vi "SaveImageAndDATA.vi"(6 "Array":dbl[][](array[numeric]), 7 "new picture":picture, 9 "Info":string, 10 "file name":string, 11 "folder":path) -> ()   [LabVIEW 2011]
uses:
  <vilib>/Utility/file.llb/Write To Spreadsheet File (DBL).vi
panel:
  out "before substring":string
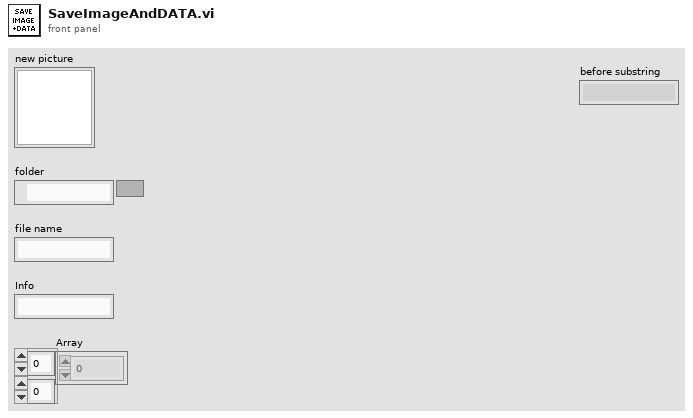
[diagram p1: front panel]
types:
  T1 = enum16{"open", "replace", "create", "open or create", "replace or create", "replace or create with confirmation"}
  T2 = typedef "imagedata.ctl" = cluster{"image type":i32, "image depth":i32, "image":u8[], "mask":u8[], "colors":u32[], "Rectangle":cluster{"left":i16, "top":i16, "right":i16, "bottom":i16}}
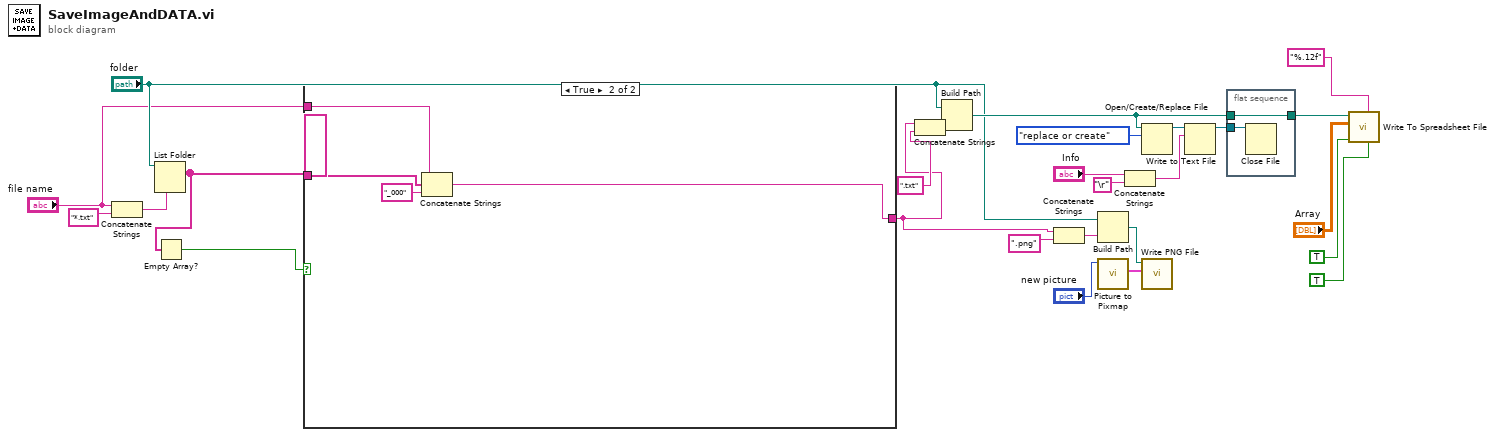
[diagram p0: block diagram]
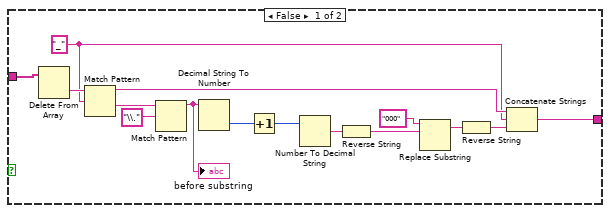
[diagram p2: hidden frame]
diagram:
  n1 = Concatenate Strings("file name", "*.txt" ("string")) -> (w22:string)
  n2 = List Folder(path="folder", pattern=w22) -> (filenames=w18:string[])  [unwired: 2 in, 3 out]
  n3 = Empty Array?(array=w18) -> (empty?=w19:bool)
  n4 = case shown="True" w19 {
    tunnel: [w41 w43] -> w20
    tunnel: w18 -> [w27 w45]
    tunnel: "file name" -> [_ w42]
    frame False {
      w29 = "_" ("regular expression")
      n5 = Delete From Array(array=w27) -> (deleted portion=w40:string)  [unwired: 2 in, 1 out]
      n6 = Match Pattern(string=w40, regular expression=w29) -> (before substring=w30:string, after substring=w39:string)  [unwired: 1 in, 2 out]
      n7 = Match Pattern(string=w39, regular expression="\\.") -> (before substring=w37:string)  [unwired: 1 in, 3 out]
      "before substring" <- w37
      n8 = Decimal String To Number(string=w37) -> (number=w36:i32)  [unwired: 2 in, 1 out]
      n9 = Increment(x=w36) -> (x+1=w35:i32)
      n10 = Number To Decimal String(number=w35) -> (decimal integer string=w34:string)  [unwired: 1 in]
      n11 = Reverse String(1:w34) -> (0:w32:string)
      n12 = Replace Substring(4:w32, 5:"000") -> (1:w31:string)  [unwired: 2 in, 1 out]
      n13 = Reverse String(1:w31) -> (0:w28:string)
      n14 = Concatenate Strings(w30, w29, w28) -> (w41:string)
    }
    frame True {
      n15 = Concatenate Strings(w42, w45, "_000" ("string")) -> (w43:string)
    }
  }
  n16 = Concatenate Strings(w20, ".txt" ("string")) -> (w26:string)
  n17 = Build Path(base path="folder", name or relative path=w26) -> (appended path=w25:path)
  n18 = Concatenate Strings(w20, ".png" ("string")) -> (w10:string)
  n19 = Build Path(base path="folder", name or relative path=w10) -> (appended path=w11:path)
  n20 = call <vilib>:"Picture to Pixmap.vi"("picture"="new picture") -> ("image data"=w1:T2)  [unwired: 9 in, 1 out]
  n21 = Concatenate Strings("Info", "\r") -> (w15:string)
  n22 = Open/Create/Replace File(file path (use dialog)=w25, operation (0:open)=T1."replace or create") -> (refnum out=w3:refnum<file>)  [unwired: 4 in, 2 out]
  n23 = call <vilib>:"Write PNG File.vi"("image data"=w1, "path to PNG file"=w11) -> ()  [unwired: 8 in, 2 out]
  n24 = Write to Text File(file (use dialog)=w3, text=w15) -> (refnum out=w4:refnum<file>)  [unwired: 2 in, 2 out]
  n25 = flat-sequence {
    tunnel: w4 -> [w47]
    tunnel: w25 -> [w46]
    tunnel: [w46] -> w5
    frame #0 {
      n26 = Close File(refnum=w47) -> ()  [unwired: 1 in, 2 out]
    }
  }
  n27 = call-poly <vilib>:"Write To Spreadsheet File.vi"("transpose? (no:F)"=TRUE, "format (%.3f)"="%.12f", "append to file? (new file:F)"=TRUE, "2D data"="Array", "file path (dialog if empty)"=w5) -> ()  [unwired: 3 in, 1 out]
